vi "StartServer.vi"(8 "error in (no error)":errorcluster) -> (0 "error out":errorcluster)   [LabVIEW 2010, in "MonitorServer.lvlib"]
uses:
  MonitorServer.lvlib
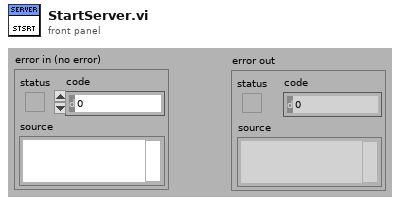
[diagram p1: front panel]
types:
  T1 = enum32{"invalid app kind", "Development System", "Run Time System", "Student Edition", "Embedded LabVIEW", "Evaluation", "Custom"}
  T2 = enum32{"Bad", "Idle", "Run top level", "Running"}
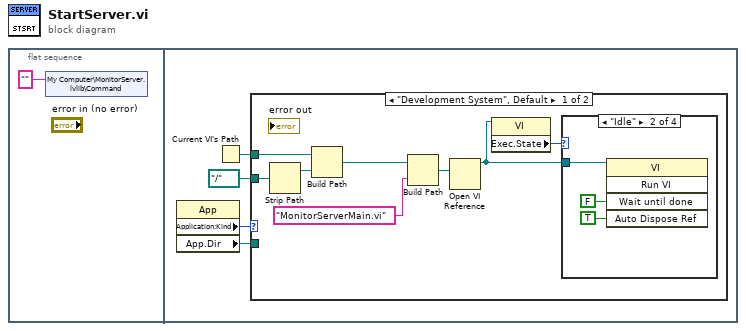
[diagram p0: block diagram]
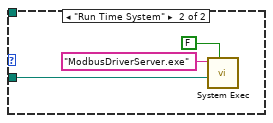
[diagram p5: hidden frame]
diagram:
  n1 = flat-sequence {
    frame #0 {
      n2 = shared-variable "My Computer\\MonitorServer.lvlib\\Command"("" ("Command")) -> ()  [unwired: 1 in, 1 out]
    }
    frame #1 {
      n3 = property class="App"() -> ("Application:Kind"=w5:T1, "App.Dir"=w2:path)  [unwired: 2 in, 2 out]
      n4 = Current VI's Path() -> (path=w3:path)
      n5 = case shown="\"Development System\", Default" w5 {
        tunnel: w3 -> [w13 _]
        tunnel: path "../.." ("relative path (.)") -> [w12 _]
        tunnel: w2 -> [_ w17]
        frame "Development System", Default {
          n6 = Strip Path(path=w12) -> (stripped path=w11:path)  [unwired: 1 out]
          n7 = Build Path(base path=w13, name or relative path=w11) -> (appended path=w10:path)
          n8 = Build Path(base path=w10, name or relative path="MonitorServerMain.vi") -> (appended path=w8:path)
          n9 = Open VI Reference(vi path=w8) -> (vi reference=w7:refnum<vi>)  [unwired: 5 in, 1 out]
          n10 = property class="VI"(reference=w7) -> ("Exec.State"=w6:T2)  [unwired: 1 in, 2 out]
          n11 = case shown="\"Idle\"" w6 {
            tunnel: w7 -> [_ w14 _ _]
            frame "Bad", Default {
            }
            frame "Idle" {
              n12 = invoke class="VI" method="Run VI"(reference=w14, "Wait until done"=FALSE ("Wait Until Done"), "Auto Dispose Ref"=TRUE ("Auto Dispose Reference")) -> ()  [unwired: 2 in, 5 out]
            }
            frame "Run top level" {
            }
            frame "Running" {
            }
          }
        }
        frame "Run Time System" {
          n13 = call <vilib>:"System Exec.vi"("wait until completion? (T)"=FALSE, "working directory"=w17, "command line"="ModbusDriverServer.exe" ("name or relative path")) -> ()  [unwired: 5 in, 4 out]
        }
      }
    }
  }
